vi "S2C_XML_CreateMeas.vi"(5 "LastTest?":bool, 7 "LastMeas?":bool, 8 "Error In":errorcluster, 10 "Result":T1, 11 "MeasData":T2) -> (0 "Error Out":errorcluster)   [LabVIEW 2015]
uses:
  S2C_XML_Globals.vi
  <vilib>/xml/Close Reference(Node).vi
  <resource>/objmgr/DOMUserDefRef.rc
  <vilib>/xml/NI_XML.lvlib
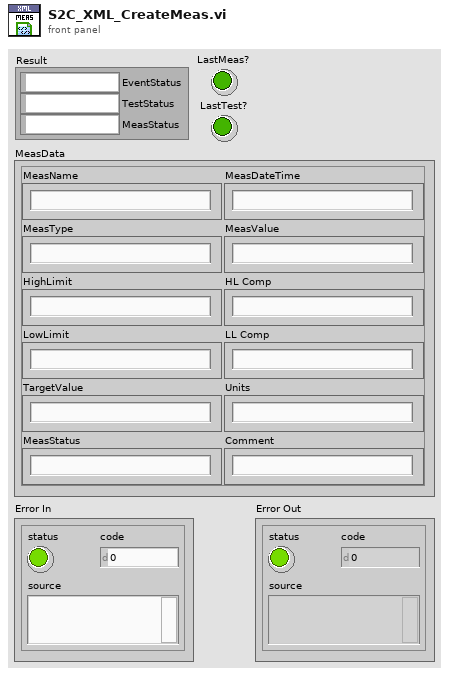
[diagram p1: front panel]
types:
  T1 = cluster{"EventStatus":string, "TestStatus":string, "MeasStatus":string}
  T2 = cluster{"MeasName":string, "MeasDateTime":string, "Comment":string, "MeasType":string, "MeasValue":string, "TargetValue":string, "HL Comp":string, "HighLimit":string, "LL Comp":string, "LowLimit":string, "Units":string, "MeasStatus":string}
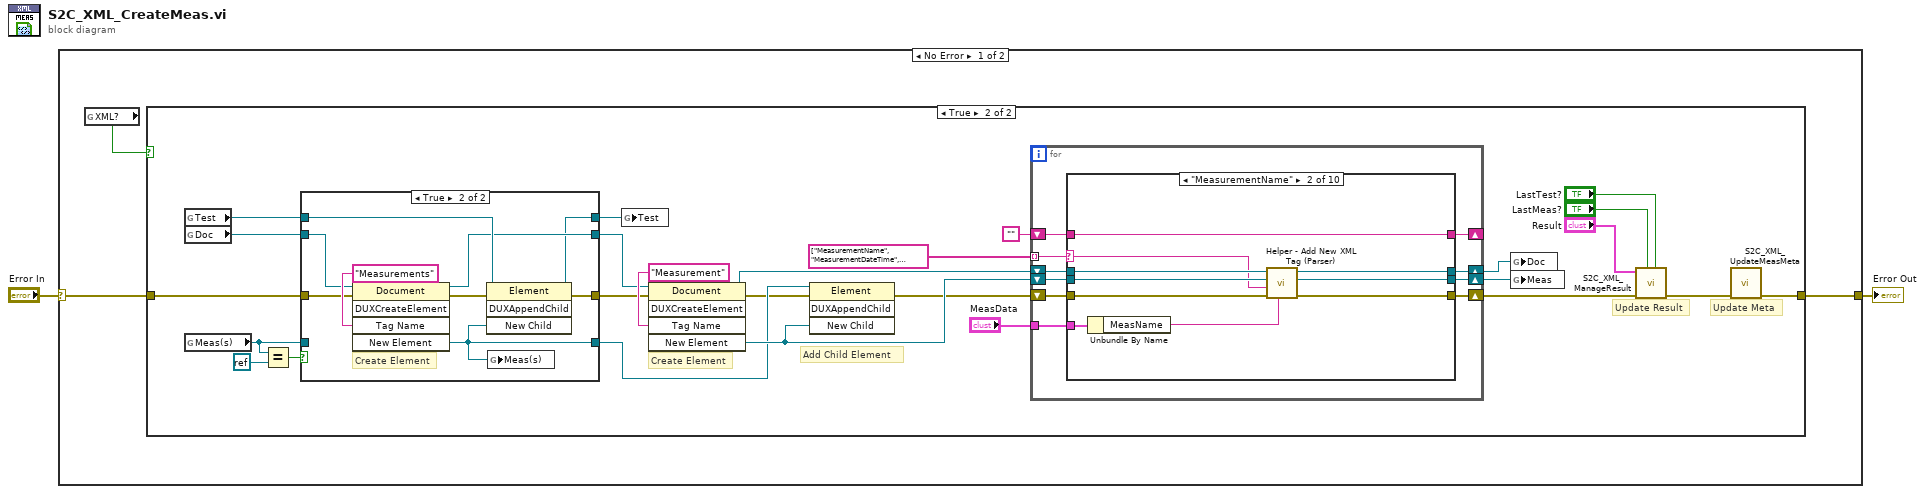
[diagram p0: block diagram]
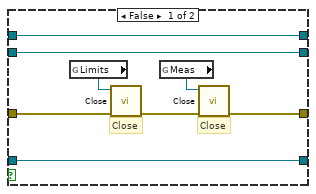
[diagram p3: hidden frame]
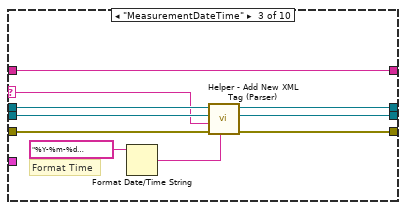
[diagram p5: hidden frame]
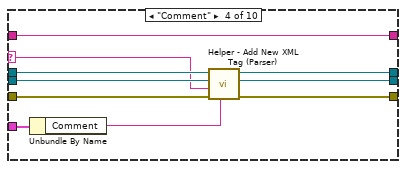
[diagram p6: hidden frame]
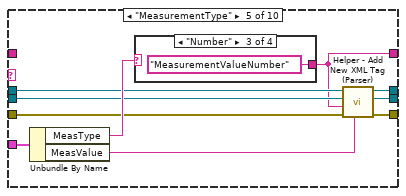
[diagram p7: hidden frame]
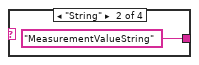
[diagram p9: hidden frame]
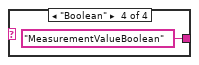
[diagram p10: hidden frame]
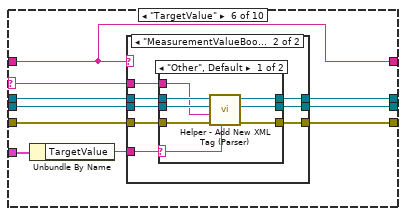
[diagram p11: hidden frame]
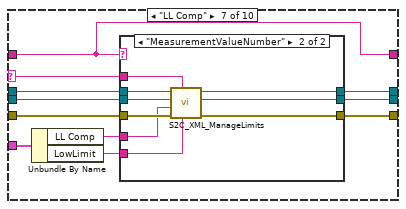
[diagram p14: hidden frame]
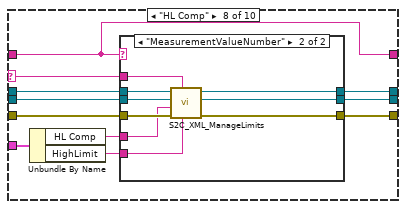
[diagram p16: hidden frame]
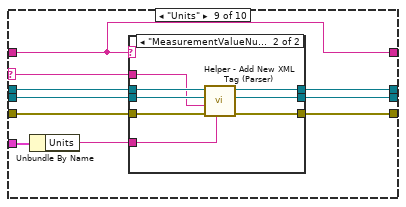
[diagram p18: hidden frame]
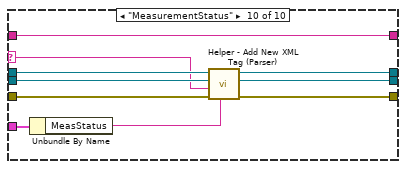
[diagram p20: hidden frame]
diagram:
  n1 = case shown="No Error" "Error In" {
    selector: "Error In" -> [w4 w216]
    tunnel: [w5 w216] -> w2
    frame No Error {
      n2 = global read "S2C_XML_Globals.vi" "XML?"() -> (w3:bool)
      n3 = case shown="True" w3 {
        tunnel: [w6 w7] -> w5
        tunnel: w4 -> [w6 w15]
        frame False {
          # "The XML Output is currently disabled"
        }
        frame True {
          # "Update Meta"
          # "Update Result"
          # "Add Child Element"
          # "Create Element"
          n4 = global read "S2C_XML_Globals.vi" "Test"() -> (w24:refnum<k20>)
          n5 = global read "S2C_XML_Globals.vi" "Doc"() -> (w18:refnum<k20>)
          n6 = global read "S2C_XML_Globals.vi" "Meas(s)"() -> (w14:refnum<k20>)
          n7 = Equal?(x=w14, y=refnum<k0> refnum) -> (x = y?=w16:bool)
          n8 = case shown="True" w16 {
            tunnel: w18 -> [w39 w48]
            tunnel: w24 -> [w40 w46]
            tunnel: [w38 w43] -> w20
            tunnel: [w40 w41] -> w23
            tunnel: [w36 w45] -> w21
            tunnel: [w39 w44] -> w22
            tunnel: w15 -> [w34 w42]
            tunnel: w14 -> [w38 _]
            frame False {
              # "Close"
              # "Close"
              n9 = global read "S2C_XML_Globals.vi" "Limits"() -> (w35:refnum<k20>)
              n10 = call-poly <vilib>:"Close.vi"("error in (no error)"=w34, "node"=w35) -> ("error out"=w33:errorcluster)  [unwired: 7 in]
              n11 = global read "S2C_XML_Globals.vi" "Meas"() -> (w37:refnum<k20>)
              n12 = call-poly <vilib>:"Close.vi"("error in (no error)"=w33, "node"=w37) -> ("error out"=w36:errorcluster)  [unwired: 7 in]
            }
            frame True {
              # "Create Element"
              n13 = invoke class="Document" method="DUXCreateElement"(reference=w48, error in=w42, "Tag Name"="Measurements") -> (reference out=w44:refnum<k20>, error out=w47:errorcluster, "New Element"=w43:refnum<k20>)  [unwired: 2 in, 2 out]
              n14 = invoke class="Element" method="DUXAppendChild"(reference=w46, error in=w47, "New Child"=w43) -> (reference out=w41:refnum<k20>, error out=w45:errorcluster)  [unwired: 1 in, 2 out]
              n15 = global write "S2C_XML_Globals.vi" "Meas(s)"(w43) -> ()
            }
          }
          n16 = global write "S2C_XML_Globals.vi" "Test"(w23) -> ()
          n17 = invoke class="Document" method="DUXCreateElement"(reference=w22, error in=w21, "Tag Name"="Measurement") -> (reference out=w28:refnum<k20>, error out=w19:errorcluster, "New Element"=w26:refnum<k20>)  [unwired: 2 in, 2 out]
          n18 = invoke class="Element" method="DUXAppendChild"(reference=w20, error in=w19, "New Child"=w26) -> (error out=w25:errorcluster)  [unwired: 1 in, 3 out]
          n19 = for {
            tunnel: string[] ["MeasurementName", "MeasurementDateTime", "Comment", "MeasurementType", "TargetValue", "LL Comp", "HL Comp", "Units", "MeasurementStatus"] -> [w58] mode=indexing
            shift-right: [w52] -> w32
            shift-left: w28 -> [w57]
            shift-right: [w53] -> w27
            shift-left: w26 -> [w56]
            shift-right: [w54] -> w9
            shift-left: w25 -> [w59]
            tunnel: "MeasData" -> [w55]
            shift-right: [w50] -> _
            shift-left: "" -> [w51]
            n20 = case shown="\"MeasurementName\"" w58 {
              selector: w58 -> [_ w66 w77 w86 _ w108 w142 w162 w187 w208]
              tunnel: w59 -> [w61 w72 w83 w92 w101 w114 w148 w171 w193 w214]
              tunnel: w57 -> [w63 w69 w80 w89 w97 w113 w147 w170 w190 w211]
              tunnel: [w63 w68 w79 w88 w99 w111 w145 w168 w189 w210] -> w52
              tunnel: w56 -> [w62 w70 w81 w90 w96 w112 w146 w169 w191 w212]
              tunnel: [w62 w67 w78 w87 w98 w110 w144 w167 w188 w209] -> w53
              tunnel: [w61 w71 w82 w91 w100 w109 w143 w166 w192 w213] -> w54
              tunnel: w55 -> [_ w73 _ w93 w103 w116 w149 w172 w194 w215]
              tunnel: w51 -> [w60 w64 w74 w84 _ w107 w139 w163 w185 w206]
              tunnel: [w60 w64 w74 w84 w94 w107 w139 w163 w185 w206] -> w50
              frame "Unknown", Default {
              }
              frame "MeasurementName" {
                n21 = Unbundle By Name(w73) -> ("MeasName"=w65:string)
                n22 = call "Helper - Add New XML Tag (Parser).vi"("Tag Data"=w65, "error in (no error)"=w72, "Tag Name"=w66, "Owning Element"=w70, "DOM document"=w69) -> ("error out"=w71:errorcluster, "dup Owning Element"=w67:refnum<k20>, "dup DOM document"=w68:refnum<k20>)  [unwired: 4 in]
              }
              frame "MeasurementDateTime" {
                # "Format Time"
                n23 = Format Date/Time String(time format string (%c)="%Y-%m-%d %H:%M:%S%3u") -> (date/time string=w75:string)  [unwired: 2 in]
                n24 = call "Helper - Add New XML Tag (Parser).vi"("Tag Data"=w75, "error in (no error)"=w83, "Tag Name"=w77, "Owning Element"=w81, "DOM document"=w80) -> ("error out"=w82:errorcluster, "dup Owning Element"=w78:refnum<k20>, "dup DOM document"=w79:refnum<k20>)  [unwired: 4 in]
              }
              frame "Comment" {
                n25 = Unbundle By Name(w93) -> ("Comment"=w85:string)
                n26 = call "Helper - Add New XML Tag (Parser).vi"("Tag Data"=w85, "error in (no error)"=w92, "Tag Name"=w86, "Owning Element"=w90, "DOM document"=w89) -> ("error out"=w91:errorcluster, "dup Owning Element"=w87:refnum<k20>, "dup DOM document"=w88:refnum<k20>)  [unwired: 4 in]
              }
              frame "MeasurementType" {
                n27 = Unbundle By Name(w103) -> ("MeasType"=w102:string, "MeasValue"=w95:string)
                n28 = case shown="\"Number\"" w102 {
                  tunnel: [_ "MeasurementValueString" "MeasurementValueNumber" "MeasurementValueBoolean"] -> w94
                  frame "Other", Default {
                  }
                  frame "String" {
                  }
                  frame "Number" {
                  }
                  frame "Boolean" {
                  }
                }
                n29 = call "Helper - Add New XML Tag (Parser).vi"("Tag Data"=w95, "error in (no error)"=w101, "Tag Name"=w94, "Owning Element"=w96, "DOM document"=w97) -> ("error out"=w100:errorcluster, "dup Owning Element"=w98:refnum<k20>, "dup DOM document"=w99:refnum<k20>)  [unwired: 4 in]
              }
              frame "TargetValue" {
                n30 = Unbundle By Name(w116) -> ("TargetValue"=w115:string)
                n31 = case shown="\"MeasurementValueBoolean\", \"MeasurementValueString\"" w107 {
                  tunnel: w115 -> [_ w127]
                  tunnel: w114 -> [w117 w126]
                  tunnel: w113 -> [w119 w125]
                  tunnel: w112 -> [w118 w124]
                  tunnel: [w119 w123] -> w111
                  tunnel: [w118 w122] -> w110
                  tunnel: [w117 w121] -> w109
                  tunnel: w108 -> [_ w120]
                  frame "Other", Default {
                  }
                  frame "MeasurementValueBoolean", "MeasurementValueString" {
                    n32 = case shown="\"Other\", Default" w127 {
                      selector: w127 -> [w129 _]
                      tunnel: w126 -> [w135 w136]
                      tunnel: w125 -> [w134 w138]
                      tunnel: w124 -> [w133 w137]
                      tunnel: [w132 w138] -> w123
                      tunnel: [w131 w137] -> w122
                      tunnel: [w130 w136] -> w121
                      tunnel: w120 -> [w128 _]
                      frame "Other", Default {
                        n33 = call "Helper - Add New XML Tag (Parser).vi"("Tag Data"=w129, "error in (no error)"=w135, "Tag Name"=w128, "Owning Element"=w133, "DOM document"=w134) -> ("error out"=w130:errorcluster, "dup Owning Element"=w131:refnum<k20>, "dup DOM document"=w132:refnum<k20>)  [unwired: 4 in]
                      }
                      frame "" {
                      }
                    }
                  }
                }
              }
              frame "LL Comp" {
                n34 = Unbundle By Name(w149) -> ("LL Comp"=w140:string, "LowLimit"=w141:string)
                n35 = case shown="\"MeasurementValueNumber\"" w139 {
                  tunnel: w148 -> [w150 w161]
                  tunnel: w147 -> [w152 w160]
                  tunnel: w146 -> [w151 w159]
                  tunnel: [w152 w158] -> w145
                  tunnel: [w151 w157] -> w144
                  tunnel: [w150 w156] -> w143
                  tunnel: w142 -> [_ w153]
                  tunnel: w141 -> [_ w155]
                  tunnel: w140 -> [_ w154]
                  frame "Other", Default {
                  }
                  frame "MeasurementValueNumber" {
                    n36 = call "S2C_XML_ManageLimits.vi"("TagValue"=w155, "Field"=w153, "Error In"=w161, "TagName"=w154, "Meas In"=w159, "Doc In"=w160) -> ("Error Out"=w156:errorcluster, "Meas Out"=w157:refnum<k20>, "Doc Out"=w158:refnum<k20>)  [unwired: 3 in]
                  }
                }
              }
              frame "HL Comp" {
                n37 = Unbundle By Name(w172) -> ("HL Comp"=w164:string, "HighLimit"=w165:string)
                n38 = case shown="\"MeasurementValueNumber\"" w163 {
                  tunnel: w171 -> [w173 w184]
                  tunnel: w170 -> [w175 w183]
                  tunnel: w169 -> [w174 w182]
                  tunnel: [w175 w181] -> w168
                  tunnel: [w174 w180] -> w167
                  tunnel: [w173 w179] -> w166
                  tunnel: w165 -> [_ w178]
                  tunnel: w164 -> [_ w177]
                  tunnel: w162 -> [_ w176]
                  frame "Other", Default {
                  }
                  frame "MeasurementValueNumber" {
                    n39 = call "S2C_XML_ManageLimits.vi"("TagValue"=w178, "Field"=w176, "Error In"=w184, "TagName"=w177, "Meas In"=w182, "Doc In"=w183) -> ("Error Out"=w179:errorcluster, "Meas Out"=w180:refnum<k20>, "Doc Out"=w181:refnum<k20>)  [unwired: 3 in]
                  }
                }
              }
              frame "Units" {
                n40 = Unbundle By Name(w194) -> ("Units"=w186:string)
                n41 = case shown="\"MeasurementValueNumber\"" w185 {
                  tunnel: w193 -> [w195 w205]
                  tunnel: [w195 w204] -> w192
                  tunnel: w191 -> [w196 w203]
                  tunnel: w190 -> [w197 w202]
                  tunnel: [w197 w201] -> w189
                  tunnel: [w196 w200] -> w188
                  tunnel: w187 -> [_ w199]
                  tunnel: w186 -> [_ w198]
                  frame "Other", Default {
                  }
                  frame "MeasurementValueNumber" {
                    n42 = call "Helper - Add New XML Tag (Parser).vi"("Tag Data"=w198, "error in (no error)"=w205, "Tag Name"=w199, "Owning Element"=w203, "DOM document"=w202) -> ("error out"=w204:errorcluster, "dup Owning Element"=w200:refnum<k20>, "dup DOM document"=w201:refnum<k20>)  [unwired: 4 in]
                  }
                }
              }
              frame "MeasurementStatus" {
                n43 = Unbundle By Name(w215) -> ("MeasStatus"=w207:string)
                n44 = call "Helper - Add New XML Tag (Parser).vi"("Tag Data"=w207, "error in (no error)"=w214, "Tag Name"=w208, "Owning Element"=w212, "DOM document"=w211) -> ("error out"=w213:errorcluster, "dup Owning Element"=w209:refnum<k20>, "dup DOM document"=w210:refnum<k20>)  [unwired: 4 in]
              }
            }
          }
          n45 = global write "S2C_XML_Globals.vi" "Doc"(w32) -> ()
          n46 = global write "S2C_XML_Globals.vi" "Meas"(w27) -> ()
          n47 = call "S2C_XML_ManageResult.vi"("LastTest?"="LastTest?", "LastMeas?"="LastMeas?", "Error In"=w9, "Result"="Result") -> ("Error Out"=w8:errorcluster)  [unwired: 7 in]
          n48 = call "S2C_XML_UpdateMeasMeta.vi"("Error In"=w8) -> ("Error Out"=w7:errorcluster)  [unwired: 10 in]
        }
      }
    }
    frame Error {
    }
  }
  "Error Out" <- w2
